vi "Video-to-Array-Convert-template and ROI.vi"() -> ()   [LabVIEW 2012]
uses:
  <vilib>/Utility/file.llb/Write To Spreadsheet File (I64).vi
panel:
  out "ROI":u8[][](array[numeric])
  in  "ROI":i32[](array[numeric])=[638, 262, 697, 321]
  out "TempBox":u8[][](array[numeric])
  in  "Frame Start":dbl=153.0
  out "Frames":T1(plugin-control)
  in  "?":bool
  in  "Template":i32[](array[numeric])=[658, 282, 677, 301]
  out "framesPerSecond":u32
  out "Image Type":T2 items=["Grayscale (U8)", "Grayscale (I16)", "Grayscale (SGL)", "Complex (CSG)", "RGB (U32)", "HSL (U32)", "RGB (U64)"]
  out "Number of Frames":u32
  in  "Path":path=path "C:/Users/admin/Desktop/lohit/pat3.avi"
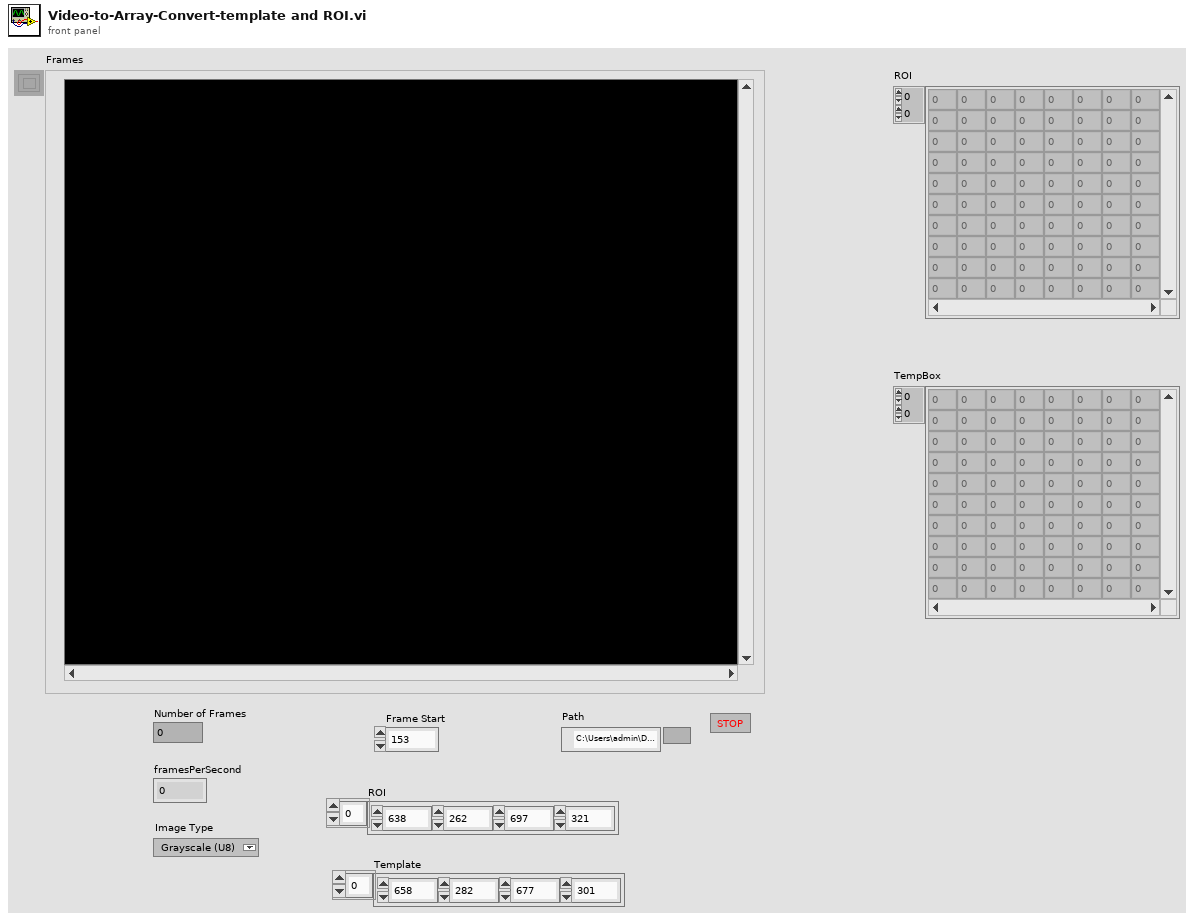
[diagram p1: front panel]
types:
  T1 = typedef "IMAQ Image.ctl" = refnum<image>
  T2 = typedef "Image Type" = u32
  T3 = typedef "AviRefnum.ctl" = refnum<k1>
  T4 = cluster{"width":u32, "height":u32, "framesPerSecond":u32, "compressionFilter":string, "hasData":bool}
  T5 = cluster{"ROI[0]":i32, "ROI[1]":i32, "ROI[2]":i32, "ROI[3]":i32, "ROI[4]":i32, "ROI[5]":i32, "ROI[6]":i32, "ROI[7]":i32, "ROI[8]":i32}
  T6 = cluster{"Template  [0]":i32, "Template  [1]":i32, "Template  [2]":i32, "Template  [3]":i32, "Template  [4]":i32, "Template  [5]":i32, "Template  [6]":i32, "Template  [7]":i32, "Template  [8]":i32}
  T7 = cluster{i32, i32, "Template  [2]":i32, "Template  [3]":i32}
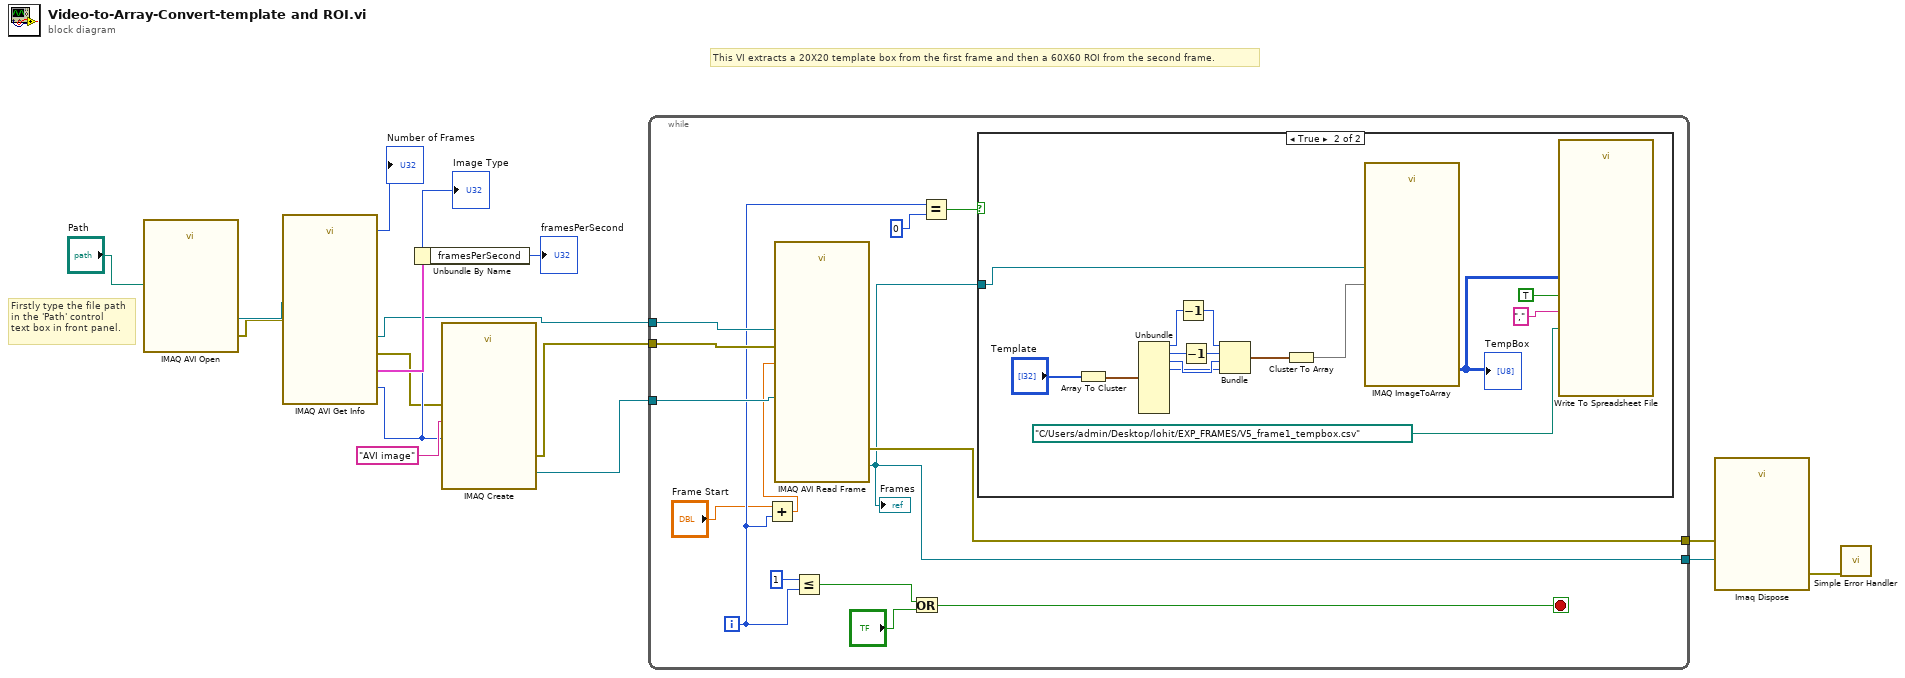
[diagram p0: block diagram]
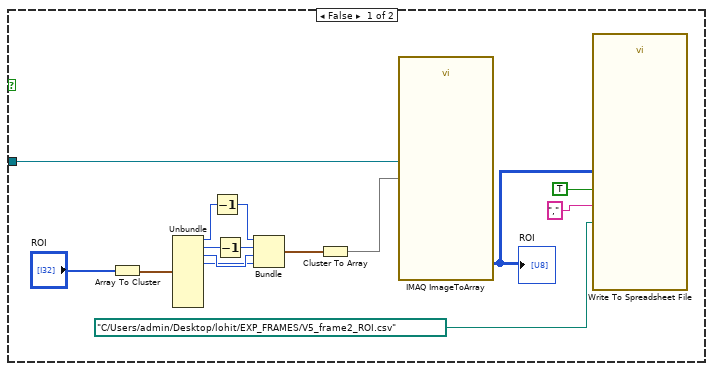
[diagram p2: hidden frame]
diagram:
  # "This VI extracts a 20X20 template box from the first frame and then a 60X60 ROI from the second frame."
  # "Firstly type the file path\nin the 'Path' control \ntext box in front panel."
  n1 = call "IMAQ AVI Open"("AVI Path"="Path") -> ("error out"=w8:errorcluster, "Avi Refnum"=w14:T3)  [unwired: 9 in]
  n2 = call "IMAQ AVI Get Info"("error in (no error)"=w8, "Avi Refnum"=w14) -> ("error out"=w7:errorcluster, "Image Type"=w10:T2, "Number of Frames"=→"Number of Frames":u32, "Avi Refnum (duplicate)"=w6:T3, "Frame Data"=w12:T4)  [unwired: 5 in]
  "Image Type" <- w10
  n3 = Unbundle By Name(w12) -> ("framesPerSecond"=→"framesPerSecond":u32)
  n4 = call "IMAQ Create"("Image Name"="AVI image", "Image Type"=w10, "error in (no error)"=w7) -> ("New Image"=w4:T1, "error out"=w5:errorcluster)  [unwired: 2 in]
  n5 = while {
    tunnel: w6 -> [w29]
    tunnel: w5 -> [w28]
    tunnel: w4 -> [w27]
    tunnel: [w16] -> w2
    tunnel: [w22] -> w1
    i -> [w19]
    stop <- w23 stop-if-true
    n6 = Add(x="Frame Start", y=w19) -> (x+y=w18:dbl)
    n7 = call "IMAQ AVI Read Frame"("error in (no error)"=w28, "Frame Number"=w18, "Image"=w27, "Avi Refnum"=w29) -> ("error out"=w22:errorcluster, "Image Out"=w16:T1)  [unwired: 4 in, 2 out]
    "Frames" <- w16
    n8 = Less Or Equal?(x=1, y=w19) -> (x <= y?=w24:bool)
    n9 = Or(x=w24, y="?") -> (x .or. y?=w23:bool)
    n10 = Equal?(x=w19, y=0) -> (x = y?=w20:bool)
    n11 = case shown="True" w20 {
      tunnel: w16 -> [w30 w57]
      frame False {
        n12 = Array To Cluster(array="ROI") -> (cluster=w40:T5)
        n13 = Unbundle "Unbundle"(w40) -> ("ROI[0]"=w39:i32, "ROI[1]"=w38:i32, "ROI[2]"=w36:i32, "ROI[3]"=w35:i32)  [unwired: 5 out]
        n14 = Decrement(x=w39) -> (x-1=w37:i32)
        n15 = Decrement(x=w38) -> (x-1=w32:i32)
        n16 = Bundle "Bundle"(w37, w32, "ROI[2]"=w36, "ROI[3]"=w35) -> (w34:cluster{i32, i32, "ROI[2]":i32, "ROI[3]":i32})  [unwired: 1 in]
        n17 = Cluster To Array(cluster=w34) -> (array=w33:i32[])
        n18 = call "IMAQ ImageToArray"("Optional Rectangle"=w33, "Image"=w30) -> ("Image Pixels (U8)"=w43:u8[][])  [unwired: 2 in, 4 out]
        "ROI" <- w43
        n19 = call-poly <vilib>:"Write To Spreadsheet File.vi"("delimiter (\\t)"="," ("delimiter (\\t)"), "append to file? (new file:F)"=TRUE, "2D data"=w43, "file path (dialog if empty)"=path "C:/Users/admin/Desktop/lohit/EXP_FRAMES/V5_frame2_ROI.csv") -> ()  [unwired: 4 in, 1 out]
      }
      frame True {
        n20 = Array To Cluster(array="Template") -> (cluster=w53:T6)
        n21 = Unbundle "Unbundle"(w53) -> ("Template  [0]"=w52:i32, "Template  [1]"=w51:i32, "Template  [2]"=w49:i32, "Template  [3]"=w48:i32)  [unwired: 5 out]
        n22 = Decrement(x=w52) -> (x-1=w50:i32)
        n23 = Decrement(x=w51) -> (x-1=w45:i32)
        n24 = Bundle "Bundle"(w50, w45, "Template  [2]"=w49, "Template  [3]"=w48) -> (w47:T7)  [unwired: 1 in]
        n25 = Cluster To Array(cluster=w47) -> (array=w46:i32[])
        n26 = call "IMAQ ImageToArray"("Optional Rectangle"=w46, "Image"=w57) -> ("Image Pixels (U8)"=w58:u8[][])  [unwired: 2 in, 4 out]
        "TempBox" <- w58
        n27 = call-poly <vilib>:"Write To Spreadsheet File.vi"("delimiter (\\t)"="," ("delimiter (\\t)"), "append to file? (new file:F)"=TRUE, "2D data"=w58, "file path (dialog if empty)"=path "C:/Users/admin/Desktop/lohit/EXP_FRAMES/V5_frame1_tempbox.csv") -> ()  [unwired: 4 in, 1 out]
      }
    }
  }
  n28 = call "Imaq Dispose"("Image"=w2, "error in (no error)"=w1) -> ("error out"=w3:errorcluster)  [unwired: 4 in]
  n29 = call <vilib>:"Simple Error Handler.vi"("error in (no error)"=w3) -> ()  [unwired: 4 in, 5 out]
